vi "Stop FGV.vi"(7 "Mode":enum16{"Set", "Get"}(ring), 8 "error in (no error)":errorcluster, 11 "Set Stop Condition":bool) -> (0 "error out (no error)":errorcluster, 3 "Get Stop Condition":bool)   [LabVIEW 2015]
doc: "Stop FGV"
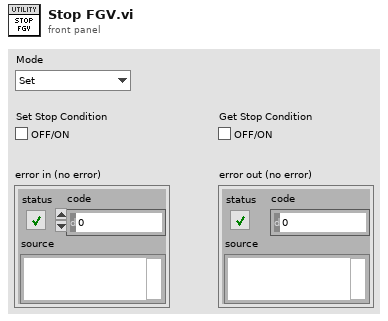
[diagram p1: front panel]
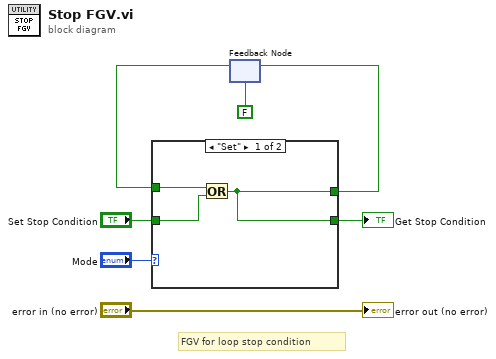
[diagram p0: block diagram]
diagram:
  # "FGV for loop stop condition"
  n1 = feedback #1(FALSE) -> (w5:bool)
  n2 = case shown="\"Set\"" "Mode" {
    tunnel: w5 -> [w10 w11]
    tunnel: [w8 w11] -> w4
    tunnel: "Set Stop Condition" -> [w9 _]
    tunnel: [w8 w11] -> w2
    frame "Set" {
      n3 = Or(x=w10, y=w9) -> (x .or. y?=w8:bool)
    }
    frame "Get", Default {
    }
  }
  "Get Stop Condition" <- w2
  n4 = feedback-in #1(w4) -> ()
  "error out (no error)" <- "error in (no error)"
